vi "SetBuvOutOFF (SubVI).vi"(0 "connection ID in":refnum<k5>, 5 "error in":errorcluster) -> (14 "connection ID out":refnum<k5>, 19 "error out":errorcluster)   [LabVIEW 2013]
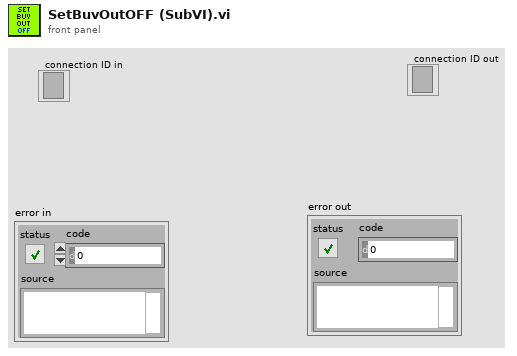
[diagram p1: front panel]
types:
  T1 = enum16{"Standard", "Buffered", "CRLF", "Immediate"}
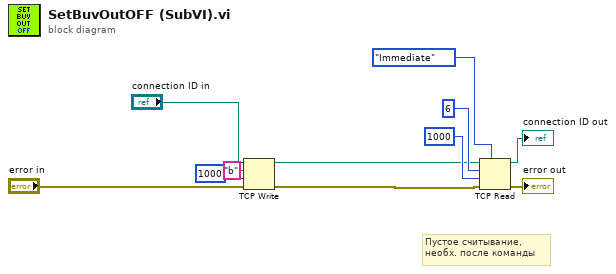
[diagram p0: block diagram]
diagram:
  # "Пустое считывание,\nнеобх. после команды"
  n1 = TCP Write(connection ID="connection ID in", data in="b", error in (no error)="error in", 9:1000 ("timeout ms (25000)")) -> (connection ID out=w1:refnum<k5>, error out=w4:errorcluster)  [unwired: 1 out]
  n2 = TCP Read(connection ID=w1, bytes to read=6, error in (no error)=w4, 7:T1."Immediate" ("mode (standard)"), 9:1000 ("timeout ms (25000)")) -> (connection ID out=→"connection ID out":refnum<k5>, error out=→"error out":errorcluster)  [unwired: 1 out]
